vi "saltos.vi"(6 "Comienza Saltos":bool=TRUE, 7 "Secuencial":bool=TRUE, 8 "Nombre Imagen":string="foto", 9 "Path":path, 10 "Parametros de Saltos":T1={"Numero de Saltos"=6, "Paso del Salto (Hz)"=100.0, "Tiempo de estabilizacion (s)"=1.0, "Frequencia de estabilizacion (Hz)"=2000.0, "Tiempo de rampa ON (s)"=5.0, "Tiempo de rampa OFF (s)"=1.0}, 11 "Numero Ultimo Experimento":i32) -> (0 "Tomando Saltos":bool=TRUE, 1 "Estable":bool=TRUE, 2 "appended path":path, 3 "Freq Output":dbl, 4 "Numero Actual Experimento":i32, 5 "Captura Imagen":bool=TRUE)   [LabVIEW 2010]
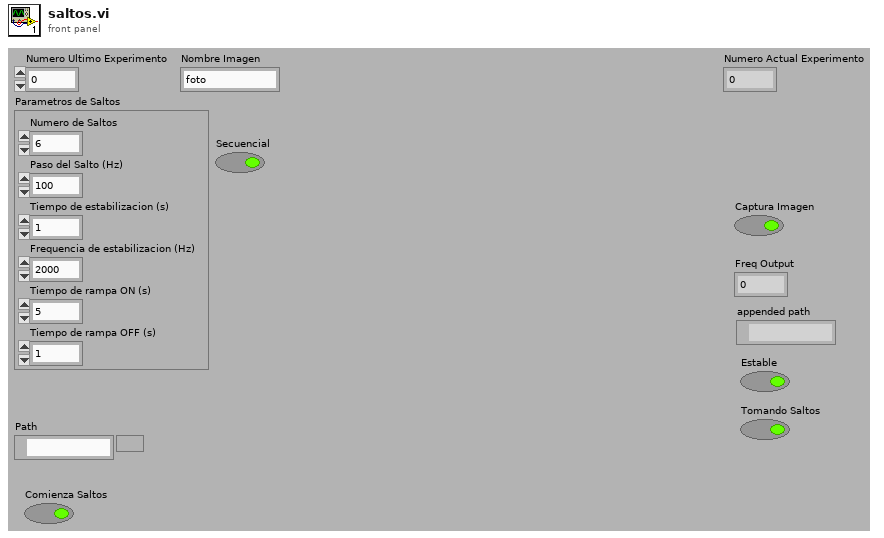
[diagram p1: front panel]
types:
  T1 = cluster{"Numero de Saltos":i32, "Paso del Salto (Hz)":dbl, "Tiempo de estabilizacion (s)":dbl, "Frequencia de estabilizacion (Hz)":dbl, "Tiempo de rampa ON (s)":dbl, "Tiempo de rampa OFF (s)":dbl}
  T2 = enum16{"Rampa ON", "Saltos", "Espera", "Toma Imagen", "Estable", "Rampa OFF", "Espera Estable"}
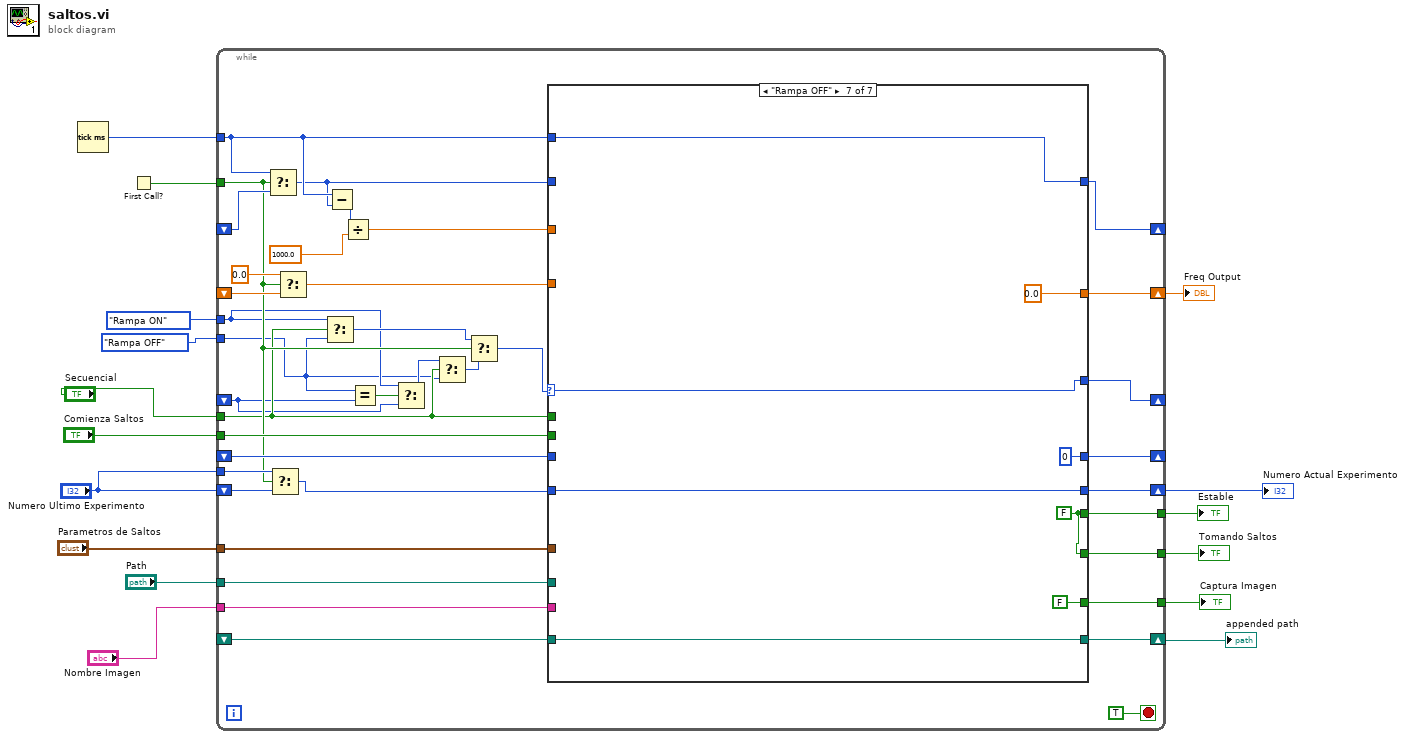
[diagram p0: block diagram]
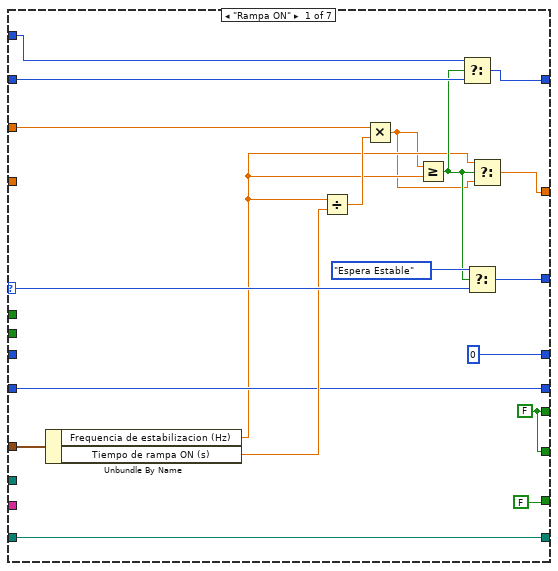
[diagram p2: hidden frame]
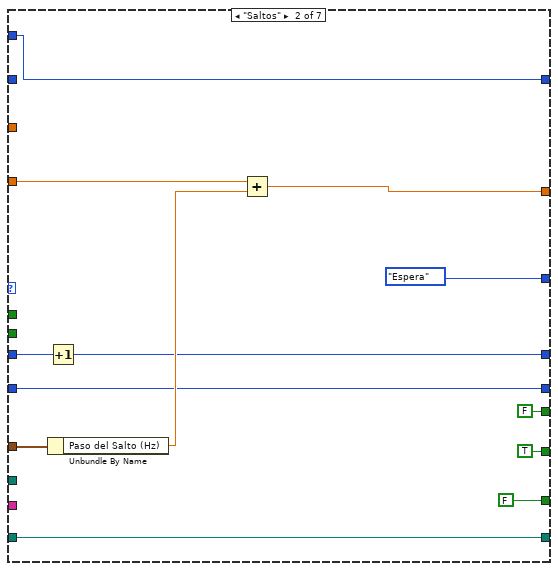
[diagram p3: hidden frame]
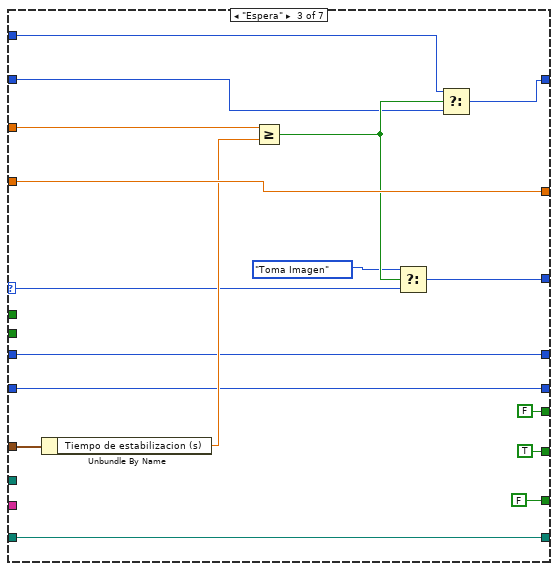
[diagram p4: hidden frame]
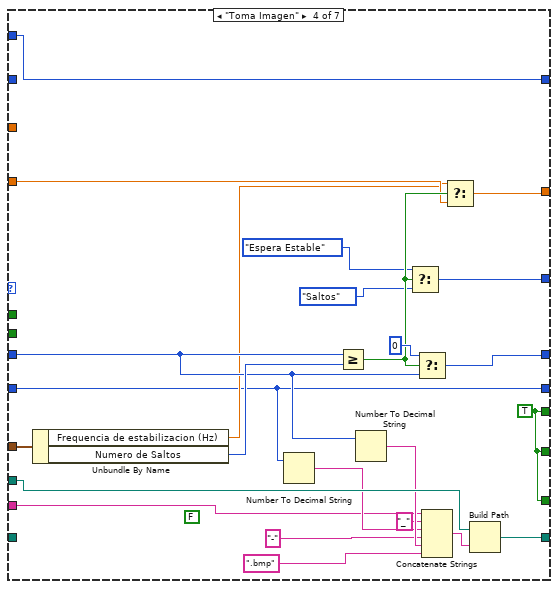
[diagram p5: hidden frame]
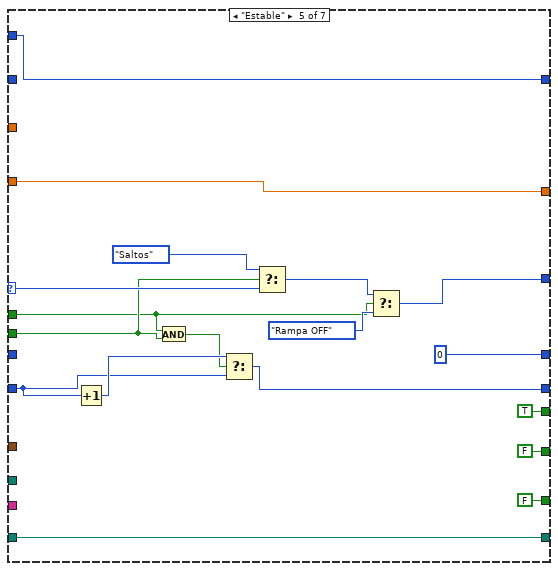
[diagram p6: hidden frame]
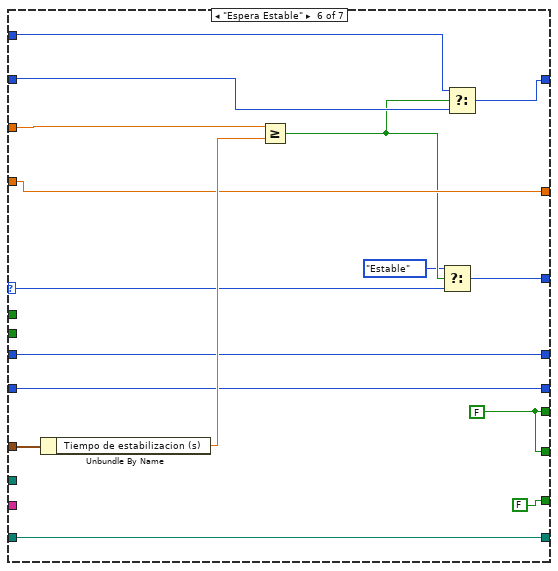
[diagram p7: hidden frame]
diagram:
  n1 = Tick Count (ms)() -> (millisecond timer value=w11:u32)
  n2 = First Call?() -> (First Call?: T/F=w16:bool)
  n3 = while {
    tunnel: w16 -> [w26]
    tunnel: w11 -> [w47]
    shift-right: [w53] -> _
    shift-left: _ -> [w39]
    shift-right: [w49] -> _
    shift-left: _ -> [w20]
    tunnel: "Parametros de Saltos" -> [w43]
    tunnel: "Comienza Saltos" -> [w46]
    shift-right: [w45] -> _
    shift-left: _ -> [w44]
    shift-right: [w48] -> w15
    shift-left: _ -> [w42]
    tunnel: "Path" -> [w38]
    shift-right: [w36] -> w8
    shift-left: _ -> [w35]
    tunnel: [w34] -> w10
    tunnel: [w33] -> w9
    tunnel: "Numero Ultimo Experimento" -> [w32]
    shift-right: [w31] -> w7
    shift-left: "Numero Ultimo Experimento" -> [w30]
    tunnel: [w28] -> w6
    tunnel: "Nombre Imagen" -> [w27]
    tunnel: "Secuencial" -> [w23]
    tunnel: T2."Rampa ON" -> [w21]
    tunnel: T2."Rampa OFF" -> [w18]
    stop <- TRUE stop-if-true
    n4 = Select(t=w47, s=w26, f=w39) -> (s? t:f=w37:u32)
    n5 = Select(t=w32, s=w26, f=w30) -> (s? t:f=w29:i32)
    n6 = Select(t=0.0, s=w26, f=w42) -> (s? t:f=w40:dbl)
    n7 = Select(t=w21, s=w23, f=w18) -> (s? t:f=w25:T2)
    n8 = Subtract(x=w47, y=w37) -> (x-y=w52:u32)
    n9 = Divide(x=w52, y=1000.0) -> (x/y=w50:dbl)
    n10 = Equal?(x=w18, y=w20) -> (x = y?=w22:bool)
    n11 = Select(t=w21, s=w22, f=w20) -> (s? t:f=w19:T2)
    n12 = Select(t=w19, s=w23, f=w18) -> (s? t:f=w17:T2)
    n13 = Select(t=w25, s=w26, f=w17) -> (s? t:f=w24:T2)
    n14 = case shown="\"Rampa OFF\"" w24 {
      selector: w24 -> [w71 _ w98 _ w145 w153 w165]
      tunnel: [w65 w80 w96 w127 w142 w156 w169] -> w53
      tunnel: w37 -> [w66 _ w93 _ _ w160 _]
      tunnel: w50 -> [w73 _ w101 _ _ w161 _]
      tunnel: [w70 T2."Espera" w99 w124 w131 w152 w165] -> w49
      tunnel: [w55 w81 w103 w115 w143 w155 0.0 ("t")] -> w48
      tunnel: w47 -> [w64 w80 w94 w127 w142 w159 w169]
      tunnel: w46 -> [_ _ _ _ w130 _ _]
      tunnel: [0 w82 w97 w123 0 w150 u32 0 ("t")] -> w45
      tunnel: w40 -> [_ w86 w103 w116 w143 w155 _]
      tunnel: w44 -> [_ w83 w97 w120 _ w150 _]
      tunnel: w43 -> [w69 w85 w102 w126 _ w158 _]
      tunnel: w38 -> [_ _ _ w121 _ _ _]
      tunnel: [w63 w79 w92 w112 w141 w149 w166] -> w36
      tunnel: w35 -> [w63 w79 w92 _ w141 w149 w166]
      tunnel: [w61 FALSE FALSE w106 TRUE w148 w164] -> w34
      tunnel: [w61 TRUE TRUE w106 FALSE w148 w164] -> w33
      tunnel: w29 -> [w60 w75 w88 w108 w136 w147 w163]
      tunnel: [w60 w75 w88 w108 w135 w147 w163] -> w31
      tunnel: [FALSE FALSE FALSE w106 FALSE FALSE FALSE] -> w28
      tunnel: w27 -> [_ _ _ w105 _ _ _]
      tunnel: w23 -> [_ _ _ _ w129 _ _]
      frame "Rampa ON" {
        w61 = FALSE
        n15 = Unbundle By Name(w69) -> ("Frequencia de estabilizacion (Hz)"=w57:dbl, "Tiempo de rampa ON (s)"=w68:dbl)
        n16 = Divide(x=w57, y=w68) -> (x/y=w72:dbl)
        n17 = Multiply(x=w73, y=w72) -> (x*y=w56:dbl)
        n18 = Greater Or Equal?(x=w56, y=w57) -> (x >= y?=w58:bool)
        n19 = Select(t=w64, s=w58, f=w66) -> (s? t:f=w65:u32)
        n20 = Select(t=T2."Espera Estable", s=w58, f=w71) -> (s? t:f=w70:T2)
        n21 = Select(t=w57, s=w58, f=w56) -> (s? t:f=w55:dbl)
      }
      frame "Saltos" {
        n22 = Increment(x=w83) -> (x+1=w82:u32)
        n23 = Unbundle By Name(w85) -> ("Paso del Salto (Hz)"=w84:dbl)
        n24 = Add(x=w86, y=w84) -> (x+y=w81:dbl)
      }
      frame "Espera" {
        n25 = Unbundle By Name(w102) -> ("Tiempo de estabilizacion (s)"=w100:dbl)
        n26 = Greater Or Equal?(x=w101, y=w100) -> (x >= y?=w95:bool)
        n27 = Select(t=T2."Toma Imagen", s=w95, f=w98) -> (s? t:f=w99:T2)
        n28 = Select(t=w94, s=w95, f=w93) -> (s? t:f=w96:u32)
      }
      frame "Toma Imagen" {
        w106 = TRUE
        (unwired) FALSE ("Compress? (N)")
        n29 = Unbundle By Name(w126) -> ("Frequencia de estabilizacion (Hz)"=w113:dbl, "Numero de Saltos"=w125:i32)
        n30 = Number To Decimal String(number=w108) -> (decimal integer string=w109:string)  [unwired: 1 in]
        n31 = Greater Or Equal?(x=w120, y=w125) -> (x >= y?=w117:bool)
        n32 = Number To Decimal String(number=w120) -> (decimal integer string=w119:string)  [unwired: 1 in]
        n33 = Select(t=T2."Espera Estable", s=w117, f=T2."Saltos") -> (s? t:f=w124:T2)
        n34 = Select(t=u32 0, s=w117, f=w120) -> (s? t:f=w123:u32)
        n35 = Concatenate Strings(w105, "_" ("string"), w109, "-" ("string"), w119, ".bmp" ("string")) -> (w118:string)
        n36 = Select(t=w113, s=w117, f=w116) -> (s? t:f=w115:dbl)
        n37 = Build Path(base path=w121, name or relative path=w118) -> (appended path=w112:path)
      }
      frame "Estable" {
        n38 = Increment(x=w136) -> (x+1=w137:i32)
        n39 = And(x=w129, y=w130) -> (x .and. y?=w128:bool)
        n40 = Select(t=w137, s=w128, f=w136) -> (s? t:f=w135:i32)
        n41 = Select(t=T2."Saltos", s=w130, f=w145) -> (s? t:f=w132:T2)
        n42 = Select(t=w132, s=w129, f=T2."Rampa OFF") -> (s? t:f=w131:T2)
      }
      frame "Espera Estable" {
        w148 = FALSE
        n43 = Unbundle By Name(w158) -> ("Tiempo de estabilizacion (s)"=w157:dbl)
        n44 = Greater Or Equal?(x=w161, y=w157) -> (x >= y?=w154:bool)
        n45 = Select(t=T2."Estable", s=w154, f=w153) -> (s? t:f=w152:T2)
        n46 = Select(t=w159, s=w154, f=w160) -> (s? t:f=w156:u32)
      }
      frame "Rampa OFF" {
        w164 = FALSE
      }
    }
  }
  "Freq Output" <- w15
  "appended path" <- w8
  "Tomando Saltos" <- w9
  "Estable" <- w10
  "Captura Imagen" <- w6
  "Numero Actual Experimento" <- w7
